vi "RSZVB Marker Search.vi"(7 "Search (0: Max Search)":i32(ring) items=["Max Search", "Min Search", "Next Peak", "Peak Search >", "< Peak Search"], 8 "error in (no error)":errorcluster {"code" format="%.0x"}, 9 "Marker (1)":i32=1, 10 "Channel (Trace) (1)":i32=1, 11 "VISA session":refnum<visa-resource-name>) -> (0 "error out":errorcluster {"code" format="%.0x"}, 3 "dup VISA session":refnum<visa-resource-name>)   [LabVIEW 2011]
doc: "This VI search with the active marker for specific points on the trace.\n\nNote(s):\n\nThe marker must be created before using CALCulate<Ch/Tr>:MARKer<Mk>[:STATe] ON.\n\nRemote-control command(s):\nCALCulate<Ch/Tr>:MARKer<Mk>:FUNCtion:EXECute MAXimum | MINimum | NPEak | RPEak | LPEak"
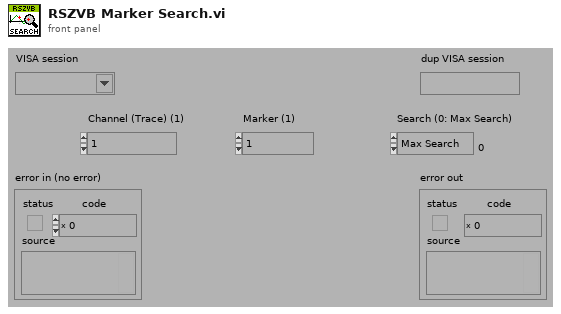
[diagram p1: front panel]
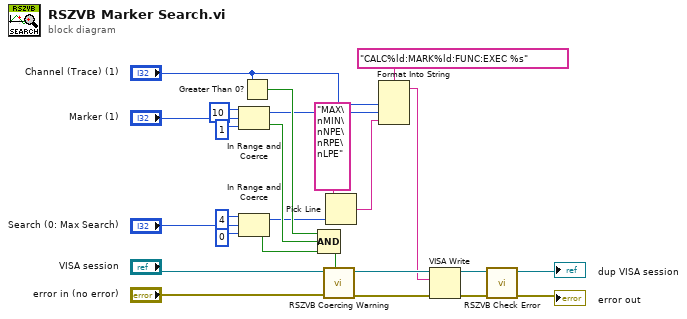
[diagram p0: block diagram]
diagram:
  n1 = In Range and Coerce(upper limit=10, x="Marker (1)", lower limit=1) -> (coerced(x)=w12:i32, In Range?=w13:bool)
  n2 = In Range and Coerce(upper limit=4, x="Search (0: Max Search)", lower limit=0) -> (coerced(x)=w8:i32, In Range?=w1:bool)
  n3 = Greater Than 0?(x="Channel (Trace) (1)") -> (x > 0?=w16:bool)
  n4 = Compound Arithmetic op=AND(w16, w13, w1) -> (w6:bool)
  n5 = call "RSZVB Coercing Warning.vi"("In Range?"=w6, "error in (no error)"="error in (no error)", "VISA session"="VISA session") -> ("error out"=w24:errorcluster, "dup VISA session"=w25:refnum<visa-resource-name>)  [unwired: 7 in]
  n6 = Pick Line(multi-line string="MAX\nMIN\nNPE\nRPE\nLPE", line index=w8) -> (output string=w7:string)  [unwired: 1 in]
  n7 = Format Into String(format string="CALC%ld:MARK%ld:FUNC:EXEC %s", "Channel (Trace) (1)", w12, w7) -> (resulting string=w5:string)  [unwired: 2 in, 1 out]
  n8 = VISA Write(VISA resource name=w25, write buffer=w5, error in (no error)=w24) -> (VISA resource name out=w22:refnum<visa-resource-name>, error out=w23:errorcluster)  [unwired: 1 out]
  n9 = call "RSZVB Check Error.vi"("error in (no error)"=w23, "VISA session"=w22) -> ("error out"=→"error out":errorcluster, "dup VISA session"=→"dup VISA session":refnum<visa-resource-name>)  [unwired: 8 in]
